vi "project.vi"() -> ()   [LabVIEW 2022 SP3]
panel:
  out "Internet OK":bool
  in  "Message":string="Hello, this message is from the host computer." caption="Recipients"
  in  "Subject":string="Message from host" caption="Recipients"
  in  "Recipients":string="someone@???.net"
  # "send email from PC"
  # "Open the block diagram for instructions"
  # "(comma separated)"
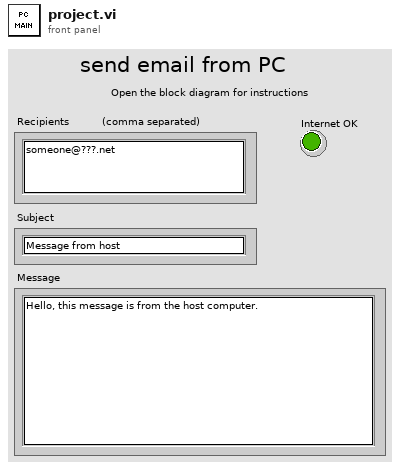
[diagram p1: front panel]
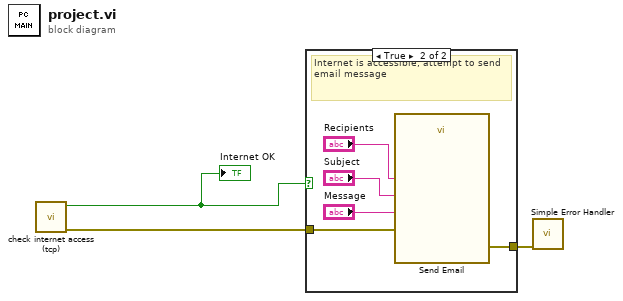
[diagram p0: block diagram]
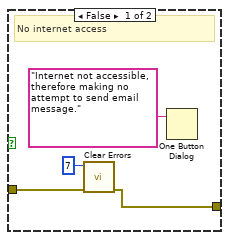
[diagram p2: hidden frame]
diagram:
  n1 = call "check internet access (tcp).vi"() -> ("error out"=w2:errorcluster, "Internet OK"=w1:bool)  [unwired: 10 in]
  "Internet OK" <- w1
  n2 = case shown="True" w1 {
    tunnel: [w4 w12] -> w3
    tunnel: w2 -> [w5 w11]
    frame False {
      # "No internet access"
      n3 = call <vilib>:"Clear Errors.vi"("error in (no error)"=w5, "specific error code to clear (0: all)"=7) -> ("error out"=w4:errorcluster)  [unwired: 4 in, 1 out]
      n4 = One Button Dialog(message="Internet not accessible, therefore making no attempt to send email message.") -> ()  [unwired: 1 in, 1 out]
    }
    frame True {
      # "Internet is accessible, attempt to send email message"
      n5 = call "Send Email"("error in"=w11, "Message"="Message", "Subject"="Subject", "Recipients"="Recipients") -> ("error out"=w12:errorcluster)  [unwired: 7 in]
    }
  }
  n6 = call <vilib>:"Simple Error Handler.vi"("error in (no error)"=w3) -> ()  [unwired: 4 in, 5 out]
